vi "Get Data SIM.vi"(8 "error in":errorcluster, 9 "Data Enqueuer":refnum<class "Message Enqueuer.lvclass">, 10 "Data":string="Simulado", 11 "SIMULATED in":refnum<class "SIMULATED.lvclass">) -> (0 "error out":errorcluster, 3 "SIMULATED out":refnum<class "SIMULATED.lvclass">)   [LabVIEW 2019, in "SIMULATED.lvclass"]
uses:
  SIMULATED.lvclass
  <vilib>/ActorFramework/Message Enqueuer/Message Enqueuer.lvclass
  Serial Devices Messages/Get Data Msg/Get Data Msg.lvclass/Get Data Msg.ctl
  <vilib>/ActorFramework/Message Enqueuer/Message Enqueuer.lvclass/Message Enqueuer.ctl
  <vilib>/ActorFramework/Message Enqueuer/Enqueue.vi
  Serial Devices Messages/Get Data Msg/Get Data Msg.lvclass
  C:/Program Files (x86)/National Instruments/LabVIEW 2019/vi.lib/ActorFramework/Message/Message.lvclass
  <vilib>/ActorFramework/Message Priority Queue/Priority Enqueue.vi
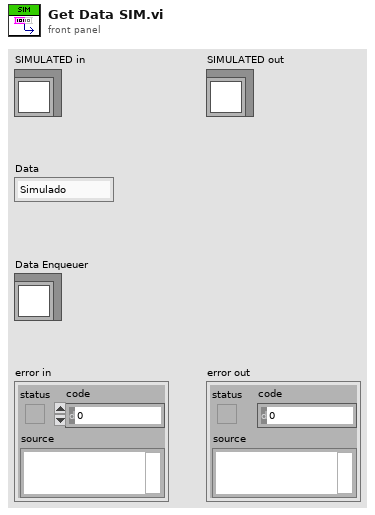
[diagram p1: front panel]
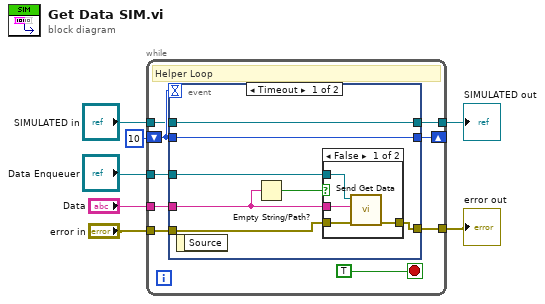
[diagram p0: block diagram]
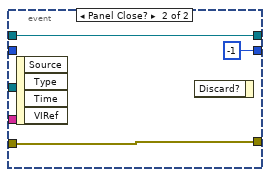
[diagram p3: hidden frame]
diagram:
  n1 = while {
    shift-right: [w16] -> _
    shift-left: 10 -> [w15]
    tunnel: "error in" -> [w14]
    tunnel: [w13] -> w6
    tunnel: "Data Enqueuer" -> [w12]
    tunnel: "SIMULATED in" -> [w11]
    tunnel: [w10] -> w2
    tunnel: "Data" -> [w8]
    stop <- TRUE stop-if-true
    # "Helper Loop"
    n2 = event shown="[0] Timeout" {
      selector: _ -> [_ _]
      dyn-events: _ -> [_ _]
      timeout: w15 -> [_ _]
      tunnel: w15 -> [w23 _]
      tunnel: [w23 -1 ("f")] -> w16
      tunnel: w14 -> [w21 w30]
      tunnel: [w20 w30] -> w13
      tunnel: w12 -> [w19 _]
      tunnel: w11 -> [w18 w29]
      tunnel: [w18 w29] -> w10
      tunnel: w8 -> [w17 _]
      event Timeout {
        n3 = event-data() -> ()  [unwired: 1 in, 1 out]
        n4 = Empty String/Path?(string/path=w17) -> (empty?=w22:bool)
        n5 = case shown="False" w22 {
          tunnel: w17 -> [w25 _]
          tunnel: w21 -> [w27 w28]
          tunnel: [w26 w28] -> w20
          tunnel: w19 -> [w24 _]
          frame False {
            n6 = call "Send Get Data.vi"("error in (no error)"=w27, "Data"=w25, "Message Enqueuer"=w24) -> ("error out"=w26:errorcluster)  [unwired: 7 in, 1 out]
          }
          frame True {
          }
        }
      }
      event Panel Close? {
        n7 = event-data() -> ()  [unwired: 1 in, 4 out]
        n8 = event-data() -> ()  [unwired: 2 in, 1 out]
      }
    }
  }
  "error out" <- w6
  "SIMULATED out" <- w2
